vi "test Import Configuration File with Parameters.vi"(8 "error in (no error)":errorcluster, 11 "TestCase in":refnum<class "Import.lvclass">) -> (0 "error out":errorcluster, 3 "TestCase out":refnum<class "Import.lvclass">)   [LabVIEW 2020, in "Import.lvclass"]
uses:
  Import.lvclass
  Shared/Port Session Configuration.ctl
  Shared/board_setup.ctl
  Shared/port_configuration.ctl
  Shared/port_setup.ctl
  Shared/tx_udp_setup.ctl
  Shared/port_tx_udp_comm.ctl
  Shared/frame_parameter.ctl
  Shared/frame_parameter_definition.ctl
  <vilib>/NI/NI VeriStand Encoding and Decoding/Encoding.ctl
  Shared/port_tx_udp_sap.ctl
  Shared/rx_udp_setup.ctl
  Shared/port_rx_udp_comm.ctl
  Shared/port_rx_udp_sap.ctl
  <vilib>/addons/_JKI Toolkits/VI Tester/TestCase.llb/TestCase.lvclass
  niveristand-custom-device-testing-tools/VeriStandTestUtilities/VeriStandTestUtilities.lvlib
  Import/AIM ARINC 664 Import.lvlib
  <vilib>/NI/NI VeriStand Encoding and Decoding/Encoding and Decoding.lvlib
  C:/Program Files (x86)/National Instruments/LabVIEW 2020/vi.lib/addons/_JKI Toolkits/VI Tester/TestCase.llb/TestCase.lvclass
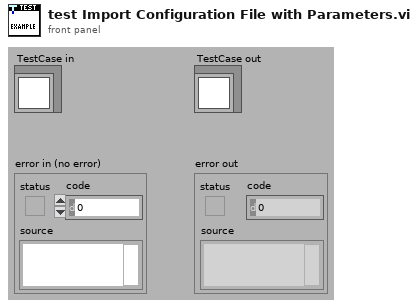
[diagram p1: front panel]
types:
  T1 = typedef "AIM ARINC 664 Import.lvlib/Port Session Configuration.ctl" = cluster{"boardSetup":T2, "portConfiguration":T3[]}
  T2 = typedef "AIM ARINC 664 Import.lvlib/board_setup.ctl" = cluster{"boardId":u32, "portSpeed":u32, "portConfig":u32}
  T3 = typedef "AIM ARINC 664 Import.lvlib/port_configuration.ctl" = cluster{"portSetup":T4, "session_tx_generic":cluster{"QueueSizeIn":u32, "count":i32, "StartMode":i32}[], "session_rx_monitor":cluster{"DefaultCronoMode":u32, "GlbMonBufferSizeIn":u32, "CaptureMode":u32, "MaxFileSizeMB":u32, "Strobe":u32, "TriggerPosition":u32}[], "Tx_UDP":cluster{"tx_udp_setup":T5, "commPorts":T6[], "sapPorts":T10[]}[], "Rx_UDP":cluster{"rx_udp_setup":T11, "commPorts":T12[], "sapPorts":T13[]}[]}
  T4 = typedef "AIM ARINC 664 Import.lvlib/port_setup.ctl" = cluster{"portId":u32, "portMap":u32}
  T5 = typedef "AIM ARINC 664 Import.lvlib/tx_udp_setup.ctl" = cluster{"VlId":i32, "Bag":i32, "NetSelect":i32, "domainID":u8, "sideID":u8, "locationID":u8, "interfaceID":u8, "NumOfSubVl":u16, "Skew":u32, "MaxFrameLength":u32, "FrameBufferSize":u32}
  T6 = typedef "AIM ARINC 664 Import.lvlib/port_tx_udp_comm.ctl" = cluster{"partitionID":u8, "UdpSrcPort":u16, "UdpDstPort":u16, "PortType":enum16{"FDX_UDP_SAMPLING", "FDX_UDP_QUEUING"}, "SubVIId":u32, "UdpNumBufMessages":u32, "UdpMaxMessageSize":u32, "UdpSamplingRate":u32, "Parameters":T7[]}
  T7 = typedef "AIM ARINC 664 Import.lvlib/frame_parameter.ctl" = cluster{"name":string, "default value":dbl, "unit":string, "Parameter":T8}
  T8 = typedef "AIM ARINC 664 Import.lvlib/frame_parameter_definition.ctl" = cluster{"start index":i32, "size":i32, "encoding":T9, "signed":bool, "scale multiplier":dbl, "scale offset":dbl}
  T9 = typedef "Encoding and Decoding.lvlib/Encoding.ctl" = enum16{"BNR", "BCD", "Discrete"}
  T10 = typedef "AIM ARINC 664 Import.lvlib/port_tx_udp_sap.ctl" = cluster{"SubVlId":u8, "UdpSrcPort":u16, "UdpNumBufMessages":u32, "UdpMaxMessageSize":u32, "partitionID":u8, "domainID":u8, "sideID":u8, "locationID":u8, "interfaceID":u8, "Parameters":T7[]}
  T11 = typedef "AIM ARINC 664 Import.lvlib/rx_udp_setup.ctl" = cluster{"VerificationMode":u32, "Bag":u32, "Jitter":u32, "MaxFrameLength":u32, "MaxSkew":u32, "VLBufSize":u32, "FilterMode":u32, "FilterPosition":u32, "Padding":u32, "FilterMask":u32, "FilterData":u32, "MinFrameLength":u32, "VlId":u16, "VLRange":u32}
  T12 = typedef "AIM ARINC 664 Import.lvlib/port_rx_udp_comm.ctl" = cluster{"domainID":u8, "sideID":u8, "locationID":u8, "partitionID":u8, "UdpSrcPort":u16, "UdpDstPort":u16, "PortType":enum16{"FDX_UDP_SAMPLING", "FDX_UDP_QUEUING"}, "SubVIId":u32, "UdpNumBufMessages":u32, "UdpMaxMessageSize":u32, "UdpSamplingRate":u32, "Parameters":T7[]}
  T13 = typedef "AIM ARINC 664 Import.lvlib/port_rx_udp_sap.ctl" = cluster{"UdpDstPort":u16, "UdpNumBufMessages":u32, "UdpMaxMessageSize":u32, "Parameters":T7[]}
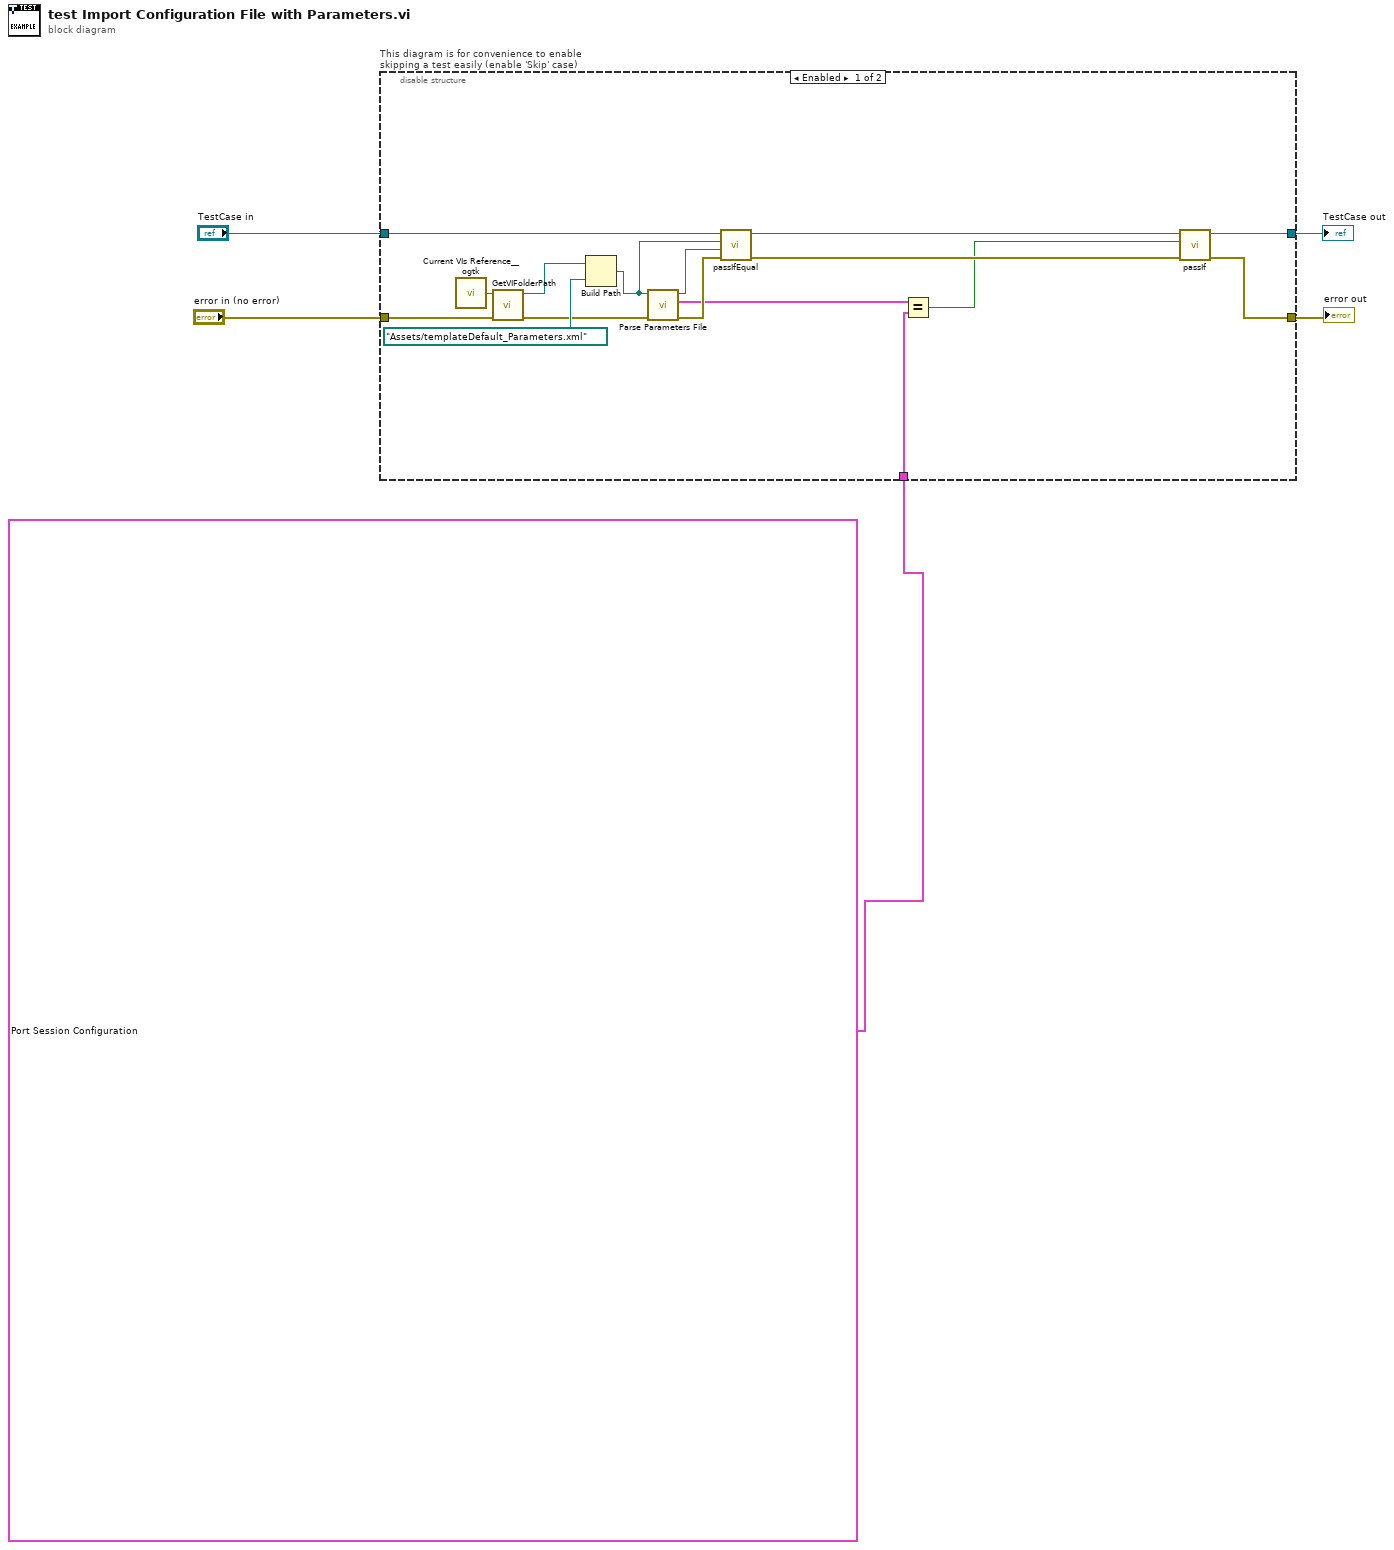
[diagram p0: block diagram]
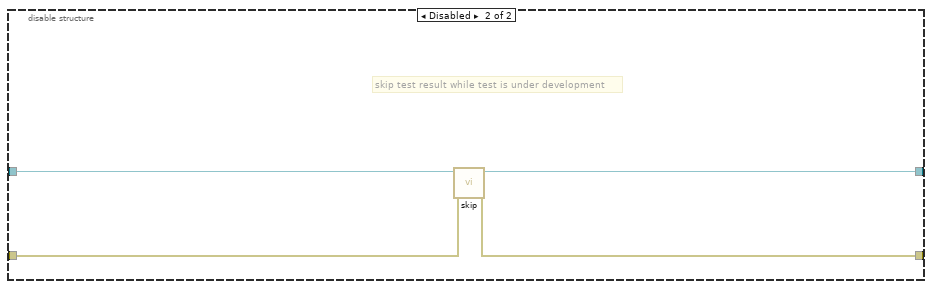
[diagram p2: hidden frame]
diagram:
  n1 = disable-structure "This diagram is for convenience to enable skipping a test easily (enable 'Skip' case)" shown="Enabled" {
    disable-tunnel: "TestCase in" -> [w14 w25]
    disable-tunnel: [w16 w23] -> w2
    disable-tunnel: [w15 w24] -> w4
    disable-tunnel: "error in (no error)" -> [w19 w22]
    disable-tunnel: T1 {"boardSetup"={"boardId"=0, "portSpeed"=0, "portConfig"=0}, "portConfiguration"=[{"portSetup"={"portId"=0, "portMap"=0}, "session_tx_generic"=[{"QueueSizeIn"=0, "count"=0, "StartMode"=1}], "session_rx_monitor"=[{"DefaultCronoMode"=1, "GlbMonBufferSizeIn"=0, "CaptureMode"=1, "MaxFileSizeMB"=1, "Strobe"=0, "TriggerPosition"=0}], "Tx_UDP"=[], "Rx_UDP"=[]}, {"portSetup"={"portId"=1, "portMap"=0}, "session_tx_generic"=[], "session_rx_monitor"=[], "Tx_UDP"=[{"tx_udp_setup"={"VlId"=0, "Bag"=1, "NetSelect"=2, "domainID"=0, "sideID"=0, "locationID"=0, "interfaceID"=0, "NumOfSubVl"=1, "Skew"=0, "MaxFrameLength"=0, "FrameBufferSize"=0}, "commPorts"=[{"partitionID"=0, "UdpSrcPort"=0, "UdpDstPort"=0, "PortType"=enum."FDX_UDP_SAMPLING", "SubVIId"=1, "UdpNumBufMessages"=0, "UdpMaxMessageSize"=0, "UdpSamplingRate"=1, "Parameters"=[{"name"="Param 0", "default value"=1.0, "unit"="fr", "Parameter"={"start index"=1, "size"=3, "encoding"=enum."BCD", "signed"=TRUE, "scale multiplier"=1.54, "scale offset"=4.0}}, {"name"="Param 1", "default value"=1.0, "unit"="fr", "Parameter"={"start index"=1, "size"=3, "encoding"=enum."BCD", "signed"=TRUE, "scale multiplier"=1.54, "scale offset"=4.0}}, {"name"="Param 2", "default value"=1.0, "unit"="fr", "Parameter"={"start index"=1, "size"=3, "encoding"=enum."BCD", "signed"=TRUE, "scale multiplier"=1.54, "scale offset"=4.0}}]}], "sapPorts"=[{"SubVlId"=1, "UdpSrcPort"=0, "UdpNumBufMessages"=0, "UdpMaxMessageSize"=0, "partitionID"=0, "domainID"=0, "sideID"=0, "locationID"=0, "interfaceID"=0, "Parameters"=[{"name"="Param 0", "default value"=1.0, "unit"="fr", "Parameter"={"start index"=1, "size"=3, "encoding"=enum."BCD", "signed"=TRUE, "scale multiplier"=1.54, "scale offset"=4.0}}, {"name"="Param 1", "default value"=1.0, "unit"="fr", "Parameter"={"start index"=1, "size"=3, "encoding"=enum."BCD", "signed"=TRUE, "scale multiplier"=1.54, "scale offset"=4.0}}, {"name"="Param 2", "default value"=1.0, "unit"="fr", "Parameter"={"start index"=1, "size"=3, "encoding"=enum."BCD", "signed"=TRUE, "scale multiplier"=1.54, "scale offset"=4.0}}]}]}], "Rx_UDP"=[{"rx_udp_setup"={"VerificationMode"=0, "Bag"=1, "Jitter"=1, "MaxFrameLength"=0, "MaxSkew"=0, "VLBufSize"=0, "FilterMode"=0, "FilterPosition"=0, "Padding"=0, "FilterMask"=0, "FilterData"=0, "MinFrameLength"=0, "VlId"=0, "VLRange"=0}, "commPorts"=[{"domainID"=0, "sideID"=0, "locationID"=0, "partitionID"=0, "UdpSrcPort"=0, "UdpDstPort"=0, "PortType"=enum."FDX_UDP_SAMPLING", "SubVIId"=0, "UdpNumBufMessages"=1, "UdpMaxMessageSize"=0, "UdpSamplingRate"=0, "Parameters"=[{"name"="Param 0", "default value"=1.0, "unit"="fr", "Parameter"={"start index"=1, "size"=3, "encoding"=enum."BCD", "signed"=TRUE, "scale multiplier"=1.54, "scale offset"=4.0}}, {"name"="Param 1", "default value"=1.0, "unit"="fr", "Parameter"={"start index"=1, "size"=3, "encoding"=enum."BCD", "signed"=TRUE, "scale multiplier"=1.54, "scale offset"=4.0}}]}], "sapPorts"=[{"UdpDstPort"=0, "UdpNumBufMessages"=0, "UdpMaxMessageSize"=0, "Parameters"=[{"name"="Param 0", "default value"=1.0, "unit"="fr", "Parameter"={"start index"=1, "size"=3, "encoding"=enum."BCD", "signed"=TRUE, "scale multiplier"=1.54, "scale offset"=4.0}}, {"name"="Param 1", "default value"=1.0, "unit"="fr", "Parameter"={"start index"=1, "size"=3, "encoding"=enum."BCD", "signed"=TRUE, "scale multiplier"=1.54, "scale offset"=4.0}}]}]}]}]} ("board configuration") -> [w6 _]
    frame Enabled {
      n2 = call <userlib>:"Current VIs Reference__ogtk.vi"() -> ("Current VI's reference"=w21:refnum<vi>)  [unwired: 5 in]
      n3 = call <vilib>:"GetVIFolderPath.vi"("error in (no error)"=w19, "VI Reference in"=w21) -> ("error out"=w17:errorcluster, "VI Folder Path out"=w20:path)  [unwired: 8 in]
      n4 = Build Path(base path=w20, name or relative path=path "Assets/templateDefault_Parameters.xml") -> (appended path=w11:path)
      n5 = call "Parse Parameters File.vi"("error in"=w17, "path to XML document"=w11) -> ("error out"=w12:errorcluster, "board configuration"=w7:T1, "path to XML document out"=w10:path)  [unwired: 7 in]
      n6 = call-dynamic "passIfEqual.vi"("error in (no error)"=w12, "y"=w10, "x"=w11, "TestCase in"=w14) -> ("error out"=w9:errorcluster, "TestCase out"=w13:refnum<class "Import.lvclass">)  [unwired: 6 in]
      n7 = Equal?(x=w7, y=w6) -> (x = y?=w8:bool)
      n8 = call-dynamic "passIf.vi"("error in (no error)"=w9, "pass"=w8, "TestCase in"=w13) -> ("error out"=w15:errorcluster, "TestCase out"=w16:refnum<class "Import.lvclass">)  [unwired: 7 in]
    }
    frame Disabled {
      # "skip test result while test is under development"
      n9 = call <vilib>:"skip.vi"("error in (no error)"=w22, "TestCase in"=w25) -> ("error out"=w24:errorcluster, "TestCase out"=w23:refnum<class "Import.lvclass">)  [unwired: 8 in]
    }
  }
  "error out" <- w4
  "TestCase out" <- w2
